vi "Set Parser Result.vi"(9 "Result":string, 10 "State":T1, 11 "Constructor String Parser In":T2) -> (3 "Constructor String Parser":T2)   [LabVIEW 2020, in "Stream.lvlib" / "URLPattern.lvclass"]
uses:
  URLPattern.lvclass
  Constructor String Parser.ctl
  Token.ctl
  Token Type.ctl
  URL Pattern Init.ctl
  Parser State.ctl
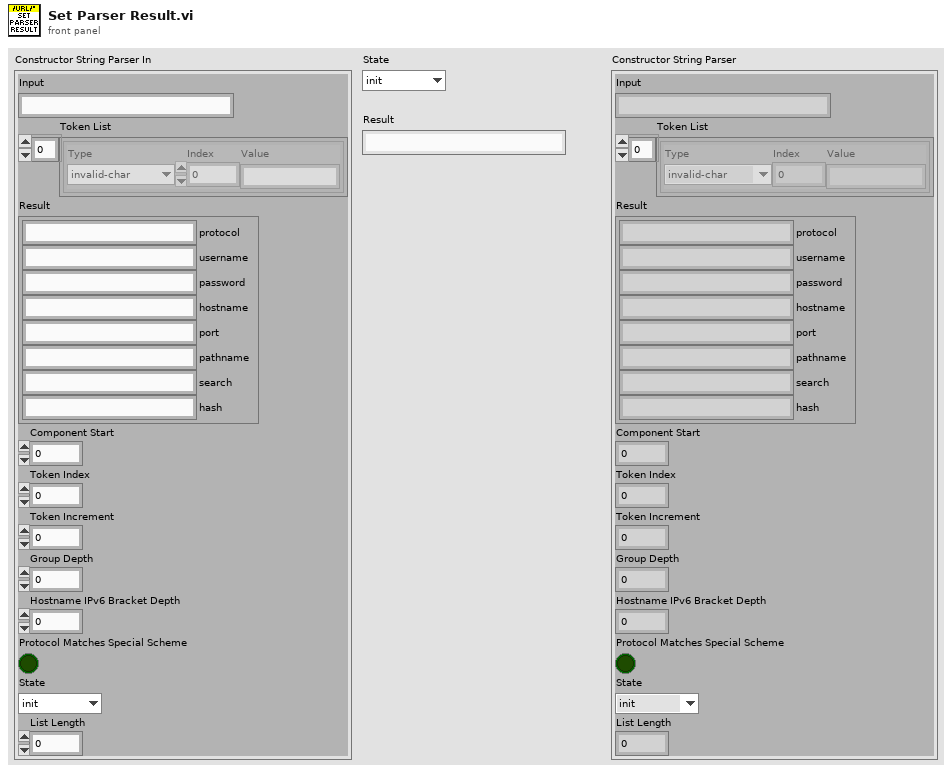
[diagram p1: front panel]
types:
  T1 = typedef "Stream.lvlib/URLPattern.lvclass/Parser State.ctl" = enum16{"init", "protocol", "authority", "username", "password", "hostname", "port", "pathname", "search", "hash", "done"}
  T2 = typedef "Stream.lvlib/URLPattern.lvclass/Constructor String Parser.ctl" = cluster{"Input":string, "Token List":T3[], "Result":T5, "Component Start":i32, "Token Index":i32, "Token Increment":i32, "Group Depth":i32, "Hostname IPv6 Bracket Depth":i32, "Protocol Matches Special Scheme":bool, "State":T1, "List Length":i32}
  T3 = typedef "Stream.lvlib/URLPattern.lvclass/Token.ctl" = cluster{"Type":T4, "Index":i32, "Value":string}
  T4 = typedef "Stream.lvlib/URLPattern.lvclass/Token Type.ctl" = enum16{"invalid-char", "open", "close", "regexp", "name", "char", "escaped-char", "other-modifier", "asterisk", "end"}
  T5 = typedef "Stream.lvlib/URLPattern.lvclass/URL Pattern Init.ctl" = cluster{"protocol":string, "username":string, "password":string, "hostname":string, "port":string, "pathname":string, "search":string, "hash":string}
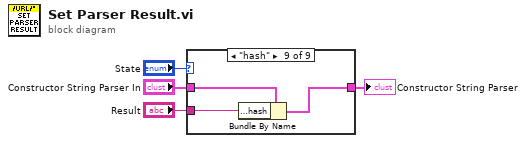
[diagram p0: block diagram]
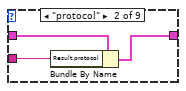
[diagram p3: hidden frame]
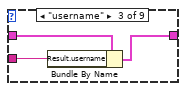
[diagram p4: hidden frame]
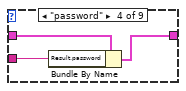
[diagram p5: hidden frame]
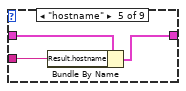
[diagram p6: hidden frame]
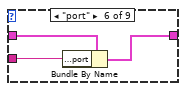
[diagram p7: hidden frame]
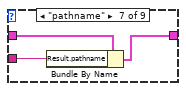
[diagram p8: hidden frame]
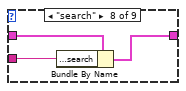
[diagram p9: hidden frame]
diagram:
  n1 = case shown="\"hash\"" "State" {
    tunnel: "Constructor String Parser In" -> [w5 w8 w11 w14 w17 w20 w23 w26 w29]
    tunnel: [w5 w7 w10 w13 w16 w19 w22 w25 w28] -> w2
    tunnel: "Result" -> [_ w6 w9 w12 w15 w18 w21 w24 w27]
    frame "init", "authority", "done" {
    }
    frame "protocol" {
      n2 = Bundle By Name(cluster=w8, "Result.protocol"=w6) -> (w7:T2)
    }
    frame "username" {
      n3 = Bundle By Name(cluster=w11, "Result.username"=w9) -> (w10:T2)
    }
    frame "password" {
      n4 = Bundle By Name(cluster=w14, "Result.password"=w12) -> (w13:T2)
    }
    frame "hostname" {
      n5 = Bundle By Name(cluster=w17, "Result.hostname"=w15) -> (w16:T2)
    }
    frame "port" {
      n6 = Bundle By Name(cluster=w20, "Result.port"=w18) -> (w19:T2)
    }
    frame "pathname" {
      n7 = Bundle By Name(cluster=w23, "Result.pathname"=w21) -> (w22:T2)
    }
    frame "search" {
      n8 = Bundle By Name(cluster=w26, "Result.search"=w24) -> (w25:T2)
    }
    frame "hash" {
      n9 = Bundle By Name(cluster=w29, "Result.hash"=w27) -> (w28:T2)
    }
  }
  "Constructor String Parser" <- w2
